vi "Legendre Polynomial_Legendre (1D).vi"(8 "type":i32(ring) items=["Standard", "Semi-Normalized", "Normalized"], 9 "m":i32, 10 "n":i32, 11 "X":dbl[](array[numeric])) -> (0 "error":i32, 3 "Legendre (n,m,X)":dbl[](array[numeric]))   [LabVIEW 2017, in "NI_AAL_Polynomial.lvlib"]
uses:
  <vilib>/Analysis/NI_AAL_Polynomial.lvlib
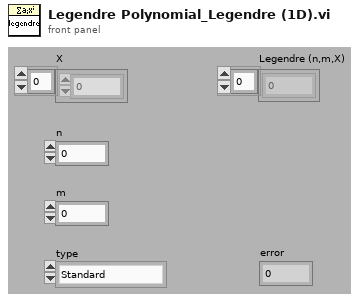
[diagram p1: front panel]
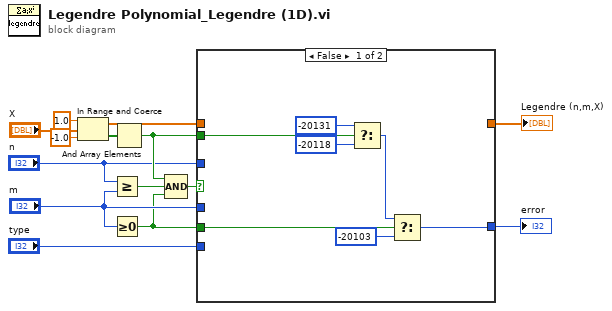
[diagram p0: block diagram]
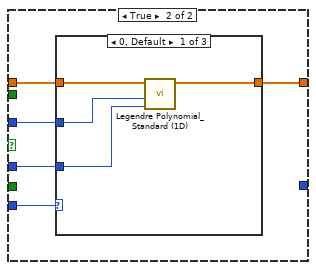
[diagram p2: hidden frame]
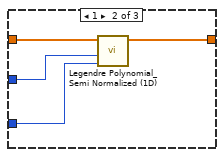
[diagram p3: hidden frame]
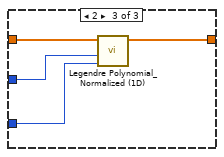
[diagram p4: hidden frame]
diagram:
  n1 = In Range and Coerce(upper limit=1.0 ("element"), x="X", lower limit=-1.0 ("element")) -> (coerced(x)=w8:dbl[], In Range?=w7:bool[])
  n2 = Greater Or Equal?(x="n", y="m") -> (x >= y?=w1:bool)
  n3 = Greater Or Equal To 0?(x="m") -> (x >= 0?=w2:bool)
  n4 = And Array Elements(Boolean array=w7) -> (logical AND=w5:bool)
  n5 = Compound Arithmetic op=AND(w5, w1, w2) -> (w6:bool)
  n6 = case shown="False" w6 {
    tunnel: w8 -> [_ w26]
    tunnel: "n" -> [_ w24]
    tunnel: "type" -> [_ w25]
    tunnel: [_ w23] -> w12
    tunnel: "m" -> [_ w22]
    tunnel: [w15 _] -> w14
    tunnel: w5 -> [w17 _]
    tunnel: w2 -> [w16 _]
    frame False {
      n7 = Select(t=-20131, s=w17, f=-20118) -> (s? t:f=w19:i32)
      n8 = Select(t=w19, s=w16, f=-20103) -> (s? t:f=w15:i32)
    }
    frame True {
      n9 = case shown="0, Default" w25 {
        tunnel: w26 -> [w28 w33 w38]
        tunnel: w22 -> [w30 w32 w35]
        tunnel: w24 -> [w29 w34 w36]
        tunnel: [w27 w31 w37] -> w23
        frame 0, Default {
          n10 = call <vilib>:"Legendre Polynomial_Standard (1D).vi"("m"=w30, "n"=w29, "X"=w28) -> ("Pnm(X)"=w27:dbl[])  [unwired: 8 out]
        }
        frame 1 {
          n11 = call <vilib>:"Legendre Polynomial_Semi Normalized (1D).vi"("m"=w32, "n"=w34, "X"=w33) -> ("Snm(X)"=w31:dbl[])  [unwired: 8 out]
        }
        frame 2 {
          n12 = call <vilib>:"Legendre Polynomial_Normalized (1D).vi"("m"=w35, "n"=w36, "X"=w38) -> ("Nnm(X)"=w37:dbl[])  [unwired: 8 out]
        }
      }
    }
  }
  "error" <- w14
  "Legendre (n,m,X)" <- w12
